vi "Execute Alphabetize Cluster Elements.vi"(6 "Mouse Position":T1, 8 "User VI Ref":refnum<vi>, 9 "Menu Item Tag Suffix":string, 10 "Remaining Items":refnum<vi>[](array[refnum]), 11 "Affected Items":T2) -> (0 "Fail transaction?":bool)   [LabVIEW 2017, in "Shortcut Menu.lvlib"]
doc: "This VI is part of a plug-in for modifying the LabVIEW shortcut menus. This is the execute VI which is called when the shortcut menu is chosen by the user. It performs the action of the selected menu item."
uses:
  Shortcut Menu.lvlib
  Alphabetize Cluster Elements.ctl
  <vilib>/Utility/miscctls.llb/LVPositionTypeDef.ctl
  Toolkit/Toolkit.lvlib
panel:
  # "All controls on this panel except \"Affected Items\" have been locked to prevent accidental edits. Changing the control names or types, other than the elements of the \"Affected Items\" cluster will make the VI unusable as a menu plugin.\n\nSee Context Help for each control for details about its use."
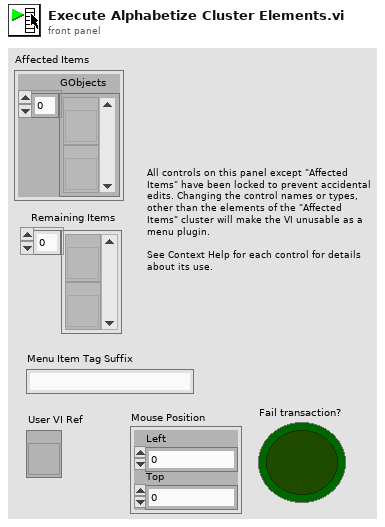
[diagram p1: front panel]
types:
  T1 = typedef "LVPositionTypeDef.ctl" = cluster{"Left":i32, "Top":i32}
  T2 = typedef "Shortcut Menu.lvlib/Alphabetize Cluster Elements.ctl" = cluster{"GObjects":refnum<vi>[]}
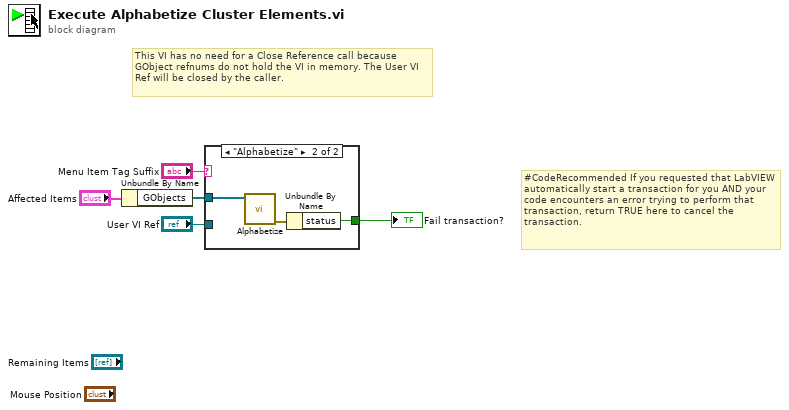
[diagram p0: block diagram]
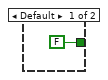
[diagram p2: hidden frame]
diagram:
  # "#CodeRecommended If you requested that LabVIEW automatically start a transaction for you AND your code encounters an error trying to perform that transaction, return TRUE here to cancel the transaction."
  # "This VI has no need for a Close Reference call because GObject refnums do not hold the VI in memory. The User VI Ref will be closed by the caller."
  n1 = Unbundle By Name("Affected Items") -> ("GObjects"=w2:refnum<vi>[])
  n2 = case shown="\"Alphabetize\"" "Menu Item Tag Suffix" {
    tunnel: [FALSE ("Fail transaction?") w9] -> w3
    tunnel: w2 -> [_ w8]
    tunnel: "User VI Ref" -> [_ _]
    frame Default {
    }
    frame "Alphabetize" {
      n3 = call "Alphabetize.vi"("Clusters In"=w8) -> ("Error Out"=w7:errorcluster)  [unwired: 8 in, 2 out]
      n4 = Unbundle By Name(w7) -> ("status"=w9:bool)
    }
  }
  "Fail transaction?" <- w3
